vi "Graph Assign Plot Names and Data.vi"(7 "Legend Number of Rows":i32, 8 "error in":errorcluster, 9 "X Ys Data":dbl[][](array[numeric]), 10 "Plot Names":string[](array[string]), 11 "Graph Ref in":refnum<vi>) -> (0 "error out":errorcluster, 2 "Plots":cluster{"Data":dbl[], "Data":dbl[]}[](array[cluster]), 3 "Graph Ref out":refnum<vi>)   [LabVIEW 2023, in "FPT_Compression UI.lvlib"]
uses:
  FPT_Compression UI.lvlib
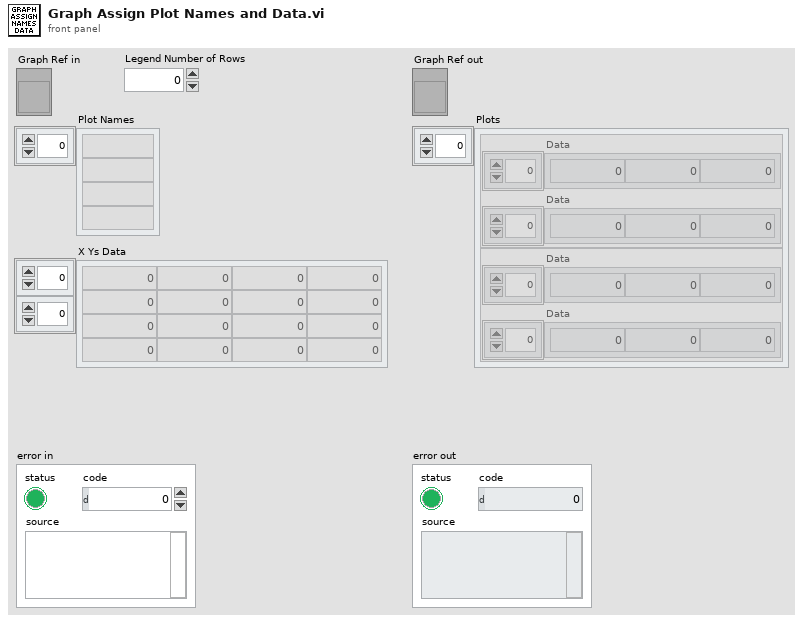
[diagram p1: front panel]
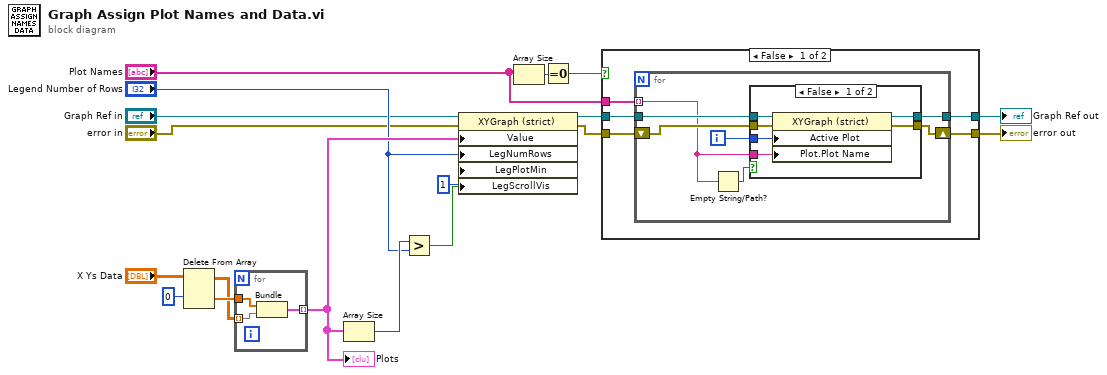
[diagram p0: block diagram]
diagram:
  n1 = Delete From Array(array="X Ys Data", index (row)=0) -> (deleted portion=w15:dbl[], array with subset deleted=w14:dbl[][])  [unwired: 2 in]
  n2 = for {
    tunnel: w15 -> [w21]
    tunnel: w14 -> [w20] mode=indexing
    tunnel: [w19] -> w10 mode=indexing
    n3 = Bundle("X Ys Data"=w21, "X Ys Data"=w20) -> (w19:cluster{"X Ys Data":dbl[], "X Ys Data":dbl[]})  [unwired: 1 in]
  }
  "Plots" <- w10
  n4 = Array Size(array=w10) -> (size(s)=w9:i32)
  n5 = Greater?(x=w9, y="Legend Number of Rows") -> (0:w7:bool)
  n6 = property on="Property Node" class="XYGraph (strict)"(reference="Graph Ref in", error in="error in", "Value"=w10, "LegNumRows"="Legend Number of Rows", "LegPlotMin"=u32 1 ("Legend:Plot Minimum"), "LegScrollVis"=w7) -> (reference out=w4:refnum<vi>, error out=w3:errorcluster)
  n7 = Array Size(array="Plot Names") -> (size(s)=w13:i32)
  n8 = Equal To 0?(x=w13) -> (x = 0?=w11:bool)
  n9 = case shown="False" w11 {
    tunnel: w3 -> [w26 w42]
    tunnel: "Plot Names" -> [w25 _]
    tunnel: w4 -> [w24 w43]
    tunnel: [w23 w43] -> w2
    tunnel: [w22 w42] -> w1
    frame False {
      n10 = for {
        tunnel: w25 -> [w27] mode=indexing
        shift-right: [w31] -> w22
        shift-left: w26 -> [w32]
        tunnel: w24 -> [w30]
        tunnel: [w29] -> w23
        i -> [w33]
        n11 = Empty String/Path?(string/path=w27) -> (empty?=w28:bool)
        n12 = case shown="False" w28 {
          tunnel: w33 -> [w39 _]
          tunnel: w27 -> [w38 _]
          tunnel: w32 -> [w37 w40]
          tunnel: [w36 w40] -> w31
          tunnel: w30 -> [w35 w41]
          tunnel: [w34 w41] -> w29
          frame False {
            n13 = property on="Property Node" class="XYGraph (strict)"(reference=w35, error in=w37, "Active Plot"=w39, "Plot.Plot Name"=w38) -> (reference out=w34:refnum<vi>, error out=w36:errorcluster)
          }
          frame True {
          }
        }
      }
    }
    frame True {
    }
  }
  "error out" <- w1
  "Graph Ref out" <- w2
